vi "Scale Picture to Centre Image.vi"(7 "Erase First? (Default: True)":bool=TRUE, 8 "error in (no error)":errorcluster, 10 "Image Size":T2, 11 "Picture in":refnum<vi>) -> (0 "error out":errorcluster, 1 "Zoom Factor Set":dbl, 3 "Draw Image to Picture Offset":T1)   [LabVIEW 2020, in "Buffer.lvclass"]
uses:
  Buffer.lvclass
  Buffer.lvclass/Buffer.ctl
  g-augmented-reality-toolkit/LabVIEW/image/Image Draw Offset.ctl
  g-augmented-reality-toolkit/LabVIEW/image/image.lvlib
  Picture Top Left Point Offset.ctl
  Image Size.ctl
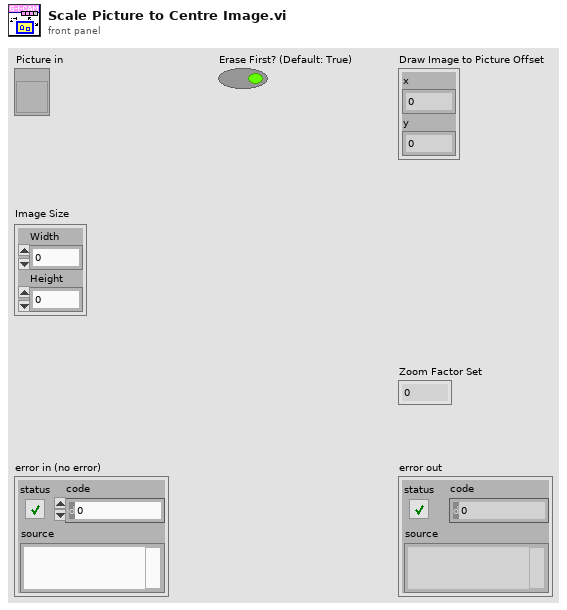
[diagram p1: front panel]
types:
  T1 = typedef "Buffer.lvclass/Picture Top Left Point Offset.ctl" = cluster{"x":i16, "y":i16}
  T2 = typedef "Buffer.lvclass/Image Size.ctl" = cluster{"Width":u16, "Height":u16}
  T3 = typedef "image.lvlib/Image Draw Offset.ctl" = cluster{"Left":i16, "Top":i16}
  T4 = typedef "LVBoundsTypeDef.ctl" = cluster{"Width":u32, "Height":u32}
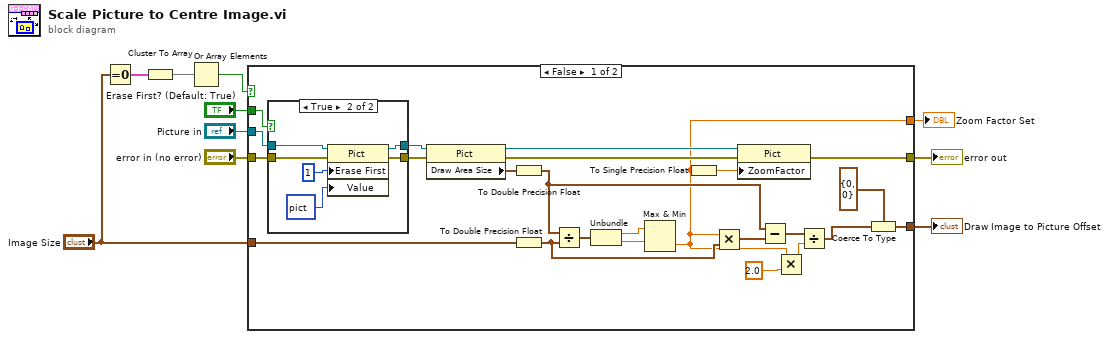
[diagram p0: block diagram]
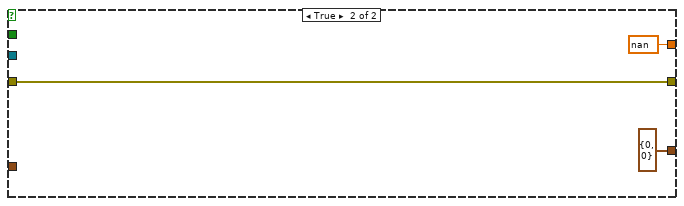
[diagram p3: hidden frame]
diagram:
  n1 = Equal To 0?(x="Image Size") -> (x = 0?=w6:cluster{"Width":bool, "Height":bool})
  n2 = Cluster To Array(cluster=w6) -> (array=w5:bool[])
  n3 = Or Array Elements(Boolean array=w5) -> (logical OR=w3:bool)
  n4 = case shown="False" w3 {
    tunnel: "Picture in" -> [w32 _]
    tunnel: "error in (no error)" -> [w31 w45]
    tunnel: [w29 T3 {"Left"=0, "Top"=0} ("Image Draw Offset (Default 0,0)")] -> w8
    tunnel: "Image Size" -> [w28 _]
    tunnel: [w27 w45] -> w4
    tunnel: "Erase First? (Default: True)" -> [w21 _]
    tunnel: [w12 nan] -> w1
    frame False {
      n5 = case shown="True" w21 {
        tunnel: [w35 w42] -> w23
        tunnel: [w36 w41] -> w26
        tunnel: w32 -> [w35 w40]
        tunnel: w31 -> [w36 w39]
        frame False {
        }
        frame True {
          n6 = property on="Property Node" class="Pict"(reference=w40, error in=w39, "Erase First"=u8 1, "Value"=picture data[5B] ("empty picture")) -> (reference out=w42:refnum<vi>, error out=w41:errorcluster)
        }
      }
      n7 = property on="Property Node" class="Pict"(reference=w23, error in=w26) -> (reference out=w22:refnum<vi>, error out=w24:errorcluster, "Draw Area Size"=w25:T4)
      n8 = To Double Precision Float(number=w25) -> (double precision float=w17:cluster{"Width":dbl, "Height":dbl})
      n9 = To Double Precision Float(number=w28) -> (double precision float=w18:cluster{"Width":dbl, "Height":dbl})
      n10 = Divide(x=w17, y=w18) -> (x/y=w34:cluster{"Width":dbl, "Height":dbl})
      n11 = Unbundle(w34) -> ("Width"=w19:dbl, "Height"=w20:dbl)
      n12 = Max & Min(x=w19, y=w20) -> (min(x,y)=w12:dbl)  [unwired: 1 out]
      n13 = To Single Precision Float(number=w12) -> (single precision float=w33:sgl)
      n14 = Multiply(x=w12, y=w18) -> (x*y=w16:cluster{"Width":dbl, "Height":dbl})
      n15 = property on="Property Node" class="Pict"(reference=w22, error in=w24, "ZoomFactor"=w33) -> (error out=w27:errorcluster)  [unwired: 1 out]
      n16 = Subtract(x=w17, y=w16) -> (x-y=w15:cluster{"Width":dbl, "Height":dbl})
      n17 = Multiply(x=w12, y=2.0) -> (x*y=w13:dbl)
      n18 = Divide(x=w15, y=w13) -> (x/y=w11:cluster{"Width":dbl, "Height":dbl})
      n19 = Coerce To Type(0:w11, 1:T1 {"x"=0, "y"=0} ("Image Draw Offset (Default 0,0)")) -> (2:w29:T1)
    }
    frame True {
    }
  }
  "Draw Image to Picture Offset" <- w8
  "error out" <- w4
  "Zoom Factor Set" <- w1
